vi "Main_Server.vi"() -> ()   [LabVIEW 2013]
uses:
  Control/TCP Multiple Connections Data.ctl
  GlobleVar/port.vi
panel:
  in  "Data":T1
  out "error out":errorcluster
  out "Message Received":string[](array[string])
  out "To Client":string
  in  "stop":bool
  out "已连接的设备数量":u32
  out "已连接的设备":string[](array[string])
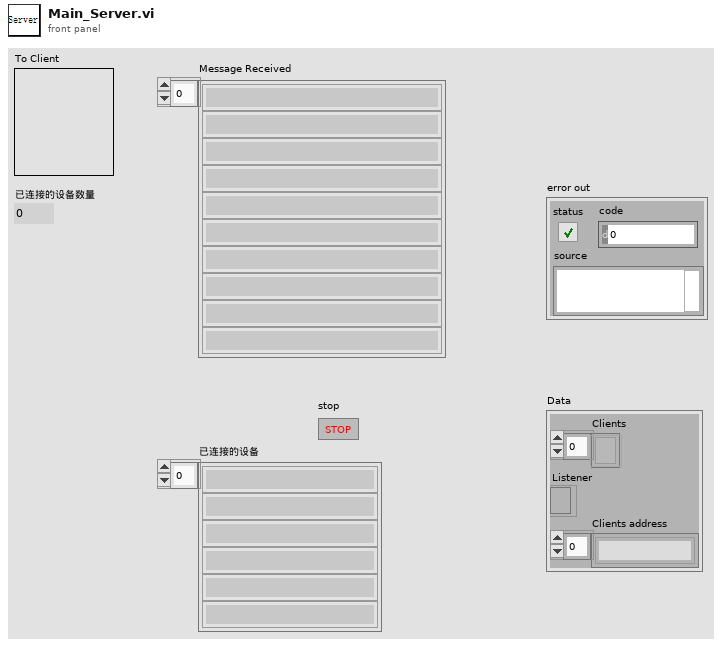
[diagram p1: front panel]
types:
  T1 = typedef "TCP Multiple Connections Data.ctl" = cluster{"Clients":refnum<k5>[], "Listener":refnum<k5>, "Clients address":string[]}
  T2 = cluster{"联机状态":bool, "外置清零信号":bool, "卡件工作模式":enum16{"无输出", "正常工作", "阀门常开", "阀门常闭"}, "卡件序列号":string, "卡件物理地址":string, "伺服阀输出电流CH1":dbl, "输出通道状态CH1":bool, "伺服阀输出电流CH2":dbl, "输出通道状态CH2":bool, "伺服输出使能CH1 ":bool, "伺服输出使能CH2":bool, "LVDT1类型":enum16{"未接入", "直流", "交流"}, "LVDT1直流回路":bool, "LVDT1次级线圈 2":bool, "LVDT1次级线圈 1":bool, "LVDT1初级线圈":bool, "LVDT2类型":enum16{"未接入", "直流", "交流"}, "LVDT2直流回路":bool, "LVDT2次级线圈 2":bool, "LVDT2次级线圈 1":bool, "LVDT2初级线圈":bool, "DEH回路状态":bool, "DEH类型":enum16{"内置", "外接"}, "转速反馈使能":bool, "LVDT1信号采样百分比":dbl, "LVDT2信号采样百分比":dbl, "DEH指令值":u8, "转速差反馈量":dbl, "回路1转速":dbl, "回路2转速":dbl, "回路3转速":dbl, "中选转速":dbl, "LVDT1 ADC":i16, "LVDT2 ADC":i16, "DEH ADC":i16, "LVDT1ZADC":i16, "LVDT2ZADC":i16, "LVDT1FADC":i16, "LVDT2FADC":i16, "DehZeroCali":bool, "DehFullCali":bool, "LVDT1ZeroCali":bool, "LVDT1FullCali":bool, "LVDT2ZeroCali":bool, "LVDT2FullCali":bool, "转速零度标定":i16, "转速满度标定":i16, "转速指令采样值":i16, "标准转速":dbl}
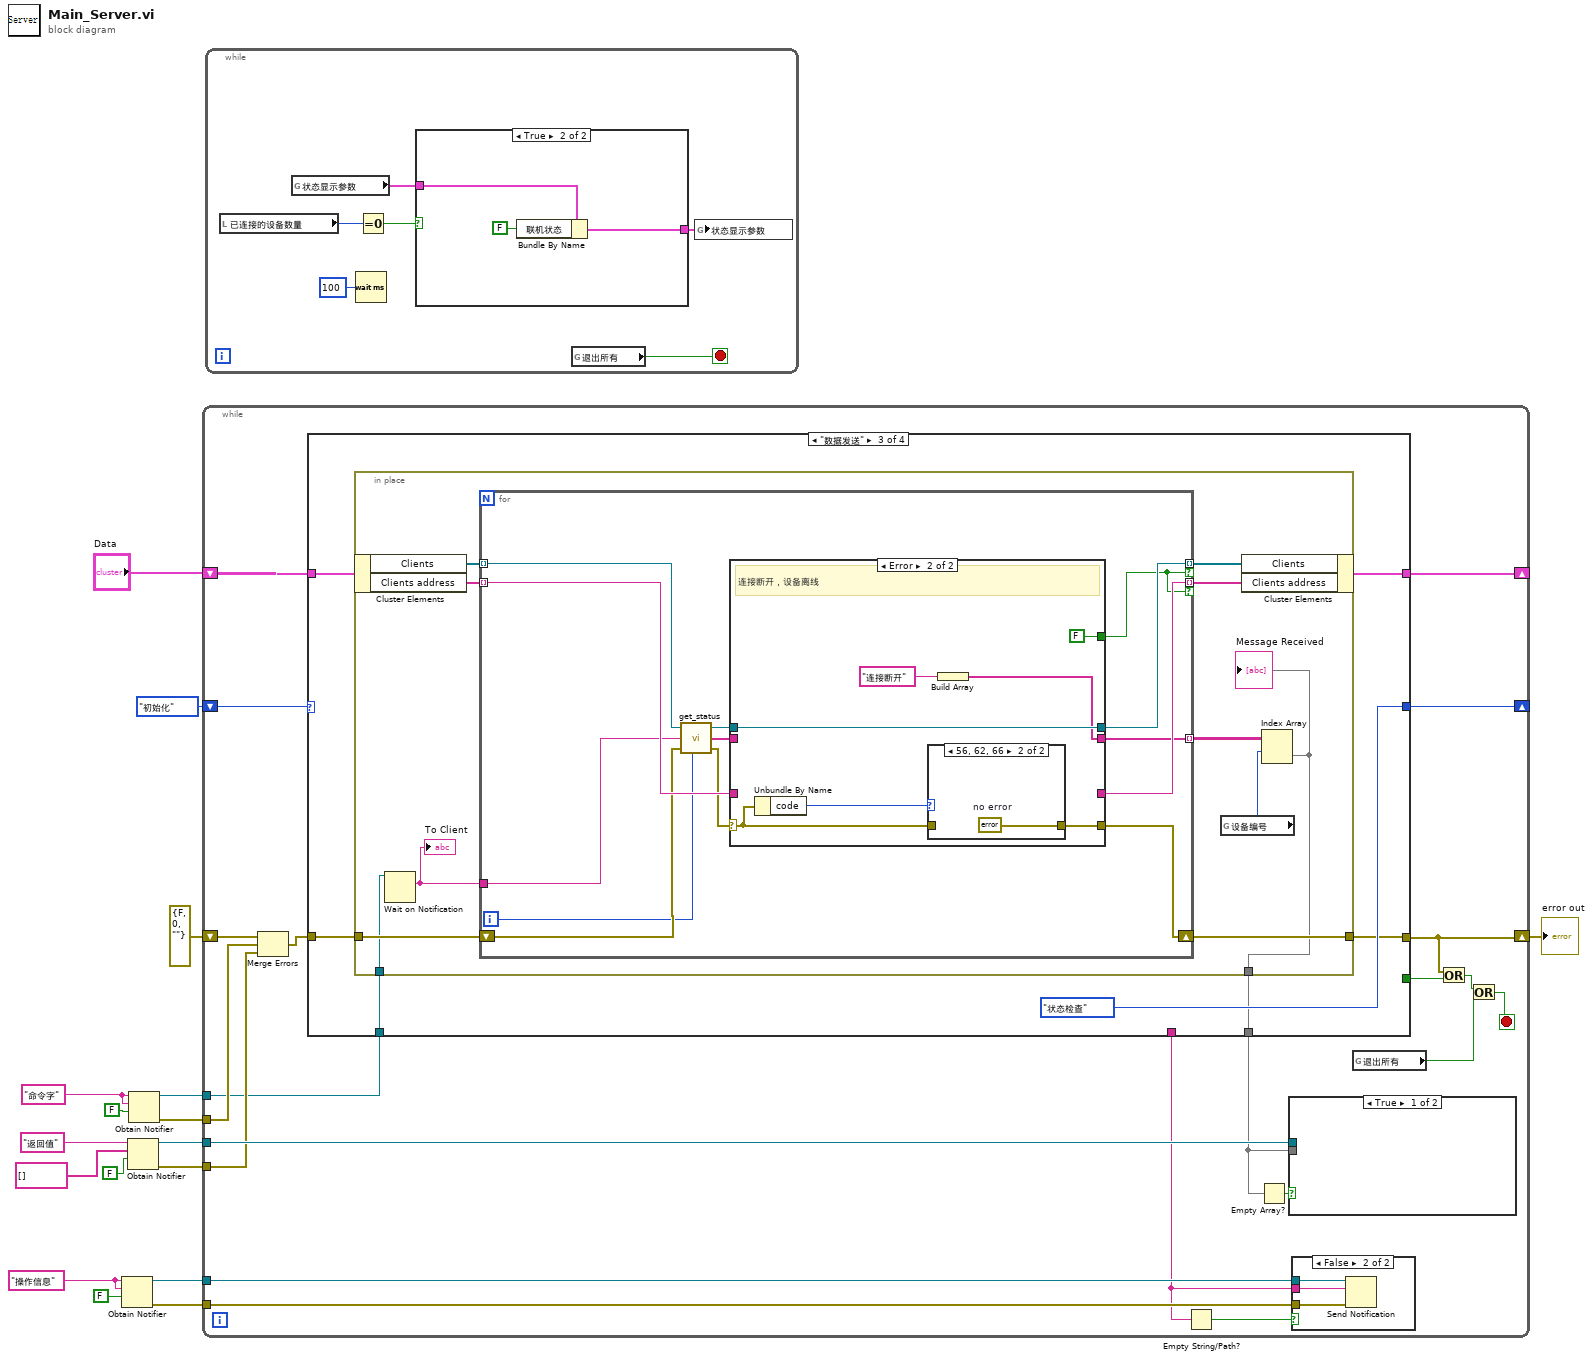
[diagram p0: block diagram]
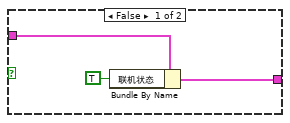
[diagram p2: hidden frame]
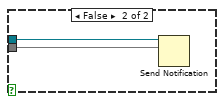
[diagram p4: hidden frame]
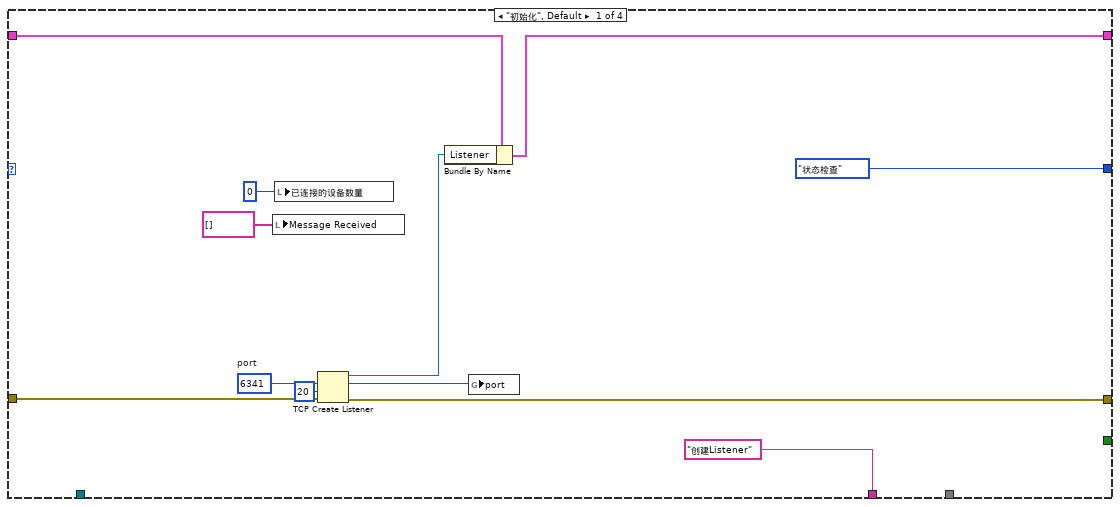
[diagram p5: hidden frame]
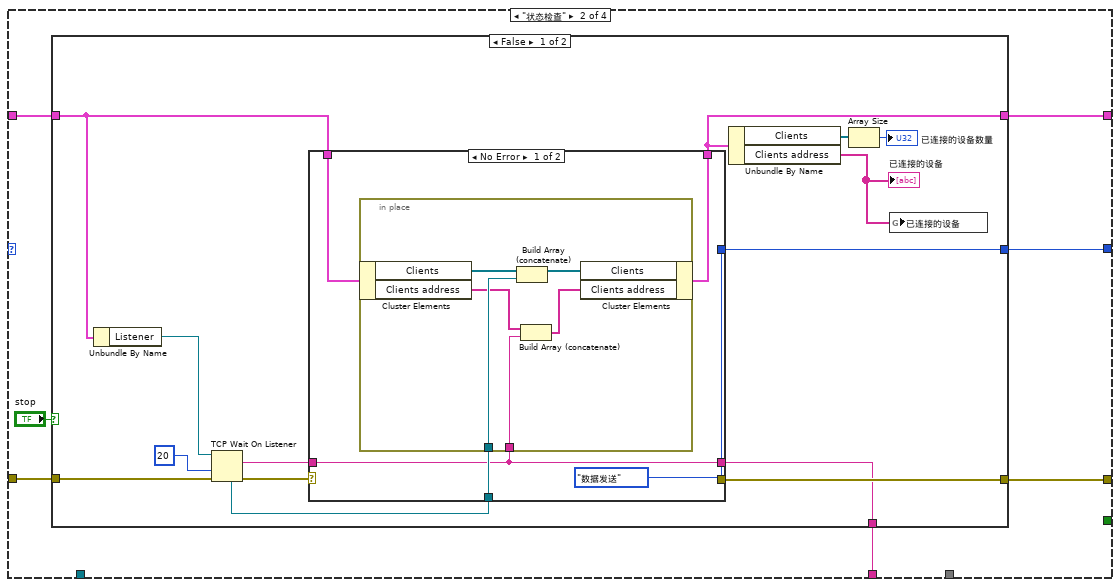
[diagram p6: hidden frame]
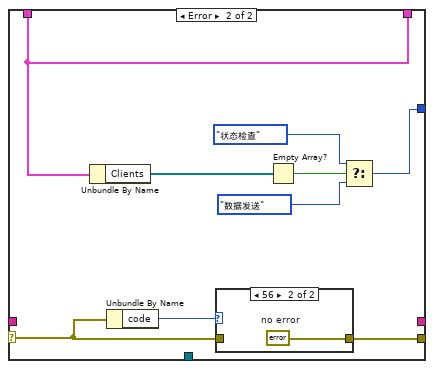
[diagram p7: hidden frame]
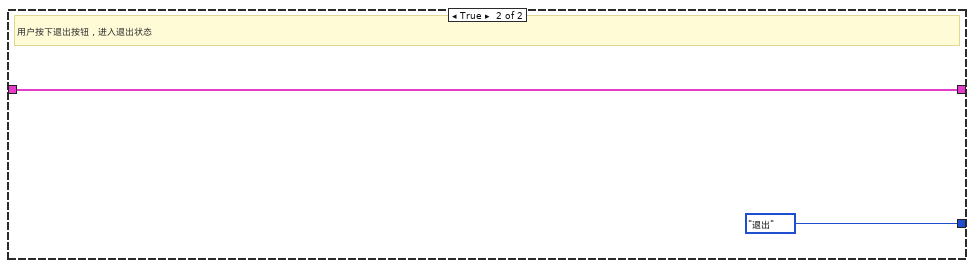
[diagram p9: hidden frame]
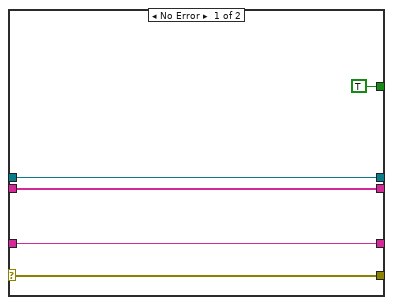
[diagram p10: hidden frame]
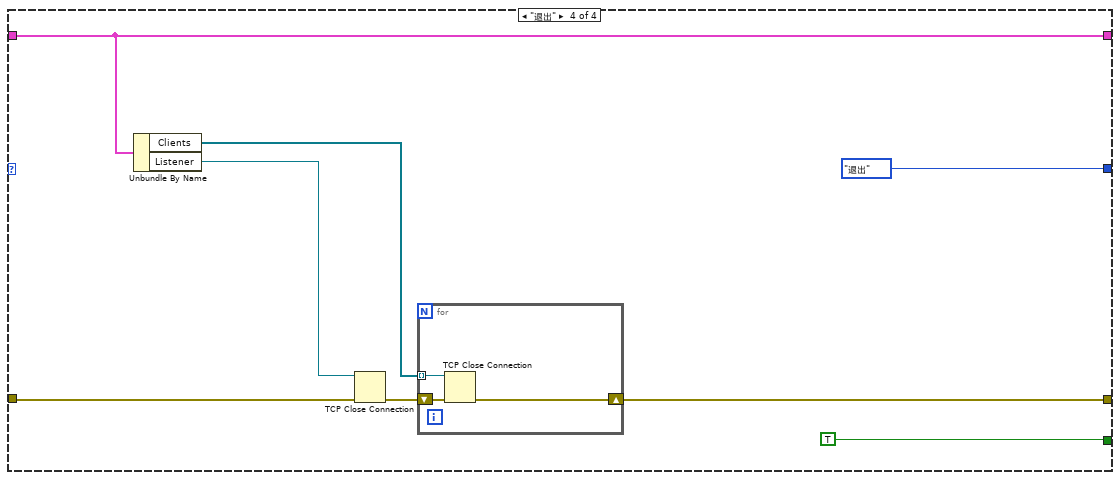
[diagram p12: hidden frame]
diagram:
  w4 = "操作信息"
  w10 = "命令字"
  n1 = Obtain Notifier(name (unnamed)=w4, notification data type=w4, create if not found? (T)=FALSE) -> (notifier out=w2:refnum<notifier>, error out=w1:errorcluster)  [unwired: 1 in, 1 out]
  n2 = Obtain Notifier(name (unnamed)="返回值", notification data type=string[] [], create if not found? (T)=FALSE) -> (notifier out=w8:refnum<notifier>, error out=w6:errorcluster)  [unwired: 1 in, 1 out]
  n3 = Obtain Notifier(name (unnamed)=w10, notification data type=w10, create if not found? (T)=FALSE) -> (notifier out=w7:refnum<notifier>, error out=w5:errorcluster)  [unwired: 1 in, 1 out]
  n4 = while {
    shift-right: [w37] -> _
    shift-left: enum16{"初始化", "状态检查", "数据发送", "退出"}."初始化" -> [w38]
    shift-right: [w33] -> _
    shift-left: "Data" -> [w36]
    shift-right: [w34] -> w14
    shift-left: errorcluster {"status"=FALSE, "code"=0, "source"=""} ("error out") -> [w26]
    tunnel: w8 -> [w31]
    tunnel: w7 -> [w18]
    tunnel: w6 -> [w23]
    tunnel: w5 -> [w25]
    tunnel: w2 -> [w21]
    tunnel: w1 -> [w20]
    stop <- w27 stop-if-true
    n5 = Merge Errors(w26, w25, w23) -> (w24:errorcluster)
    n6 = case shown="\"数据发送\"" w38 {
      tunnel: [enum16{"初始化", "状态检查", "数据发送", "退出"}."状态检查" w61 enum16{"初始化", "状态检查", "数据发送", "退出"}."状态检查" enum16{"初始化", "状态检查", "数据发送", "退出"}."退出"] -> w37
      tunnel: w24 -> [w52 w59 w104 w151]
      tunnel: [w51 w57 w103 w152] -> w34
      tunnel: w36 -> [w49 w60 w106 w147]
      tunnel: [w50 w58 w105 w147] -> w33
      tunnel: [_ _ _ TRUE] -> w35
      tunnel: [_ _ w102 _] -> w30
      tunnel: ["创建Listener" w56 _ _] -> w19
      tunnel: w18 -> [_ _ w101 _]
      frame "初始化", Default {
        w54 = u16 6341  # port
        n7 = local write "Message Received"(string[] [] ("Message Received")) -> ()
        n8 = local write "已连接的设备数量"(u32 0 ("已连接的设备数量")) -> ()
        n9 = TCP Create Listener(8:w52, 9:20 ("timeout ms (25000)"), 10:w54) -> (0:w51:errorcluster, 2:w46:u16, 3:w53:refnum<k5>)  [unwired: 2 out]
        n10 = Bundle By Name(cluster=w49, "Listener"=w53) -> (w50:T1)
        n11 = global write "port.vi" "port"(w46) -> ()
      }
      frame "状态检查" {
        n12 = case shown="False" "stop" {
          tunnel: [w69 enum16{"初始化", "状态检查", "数据发送", "退出"}."退出"] -> w61
          tunnel: w60 -> [w73 w99]
          tunnel: w59 -> [w75 _]
          tunnel: [w67 w99] -> w58
          tunnel: [w68 _] -> w57
          tunnel: [w63 _] -> w56
          frame False {
            n13 = Unbundle By Name(w73) -> ("Listener"=w76:refnum<k5>)
            n14 = TCP Wait On Listener(8:w75, 9:20 ("timeout ms (wait forever: -1)"), 11:w76) -> (0:w74:errorcluster, 2:w71:string, 4:w72:refnum<k5>)  [unwired: 1 in, 2 out]
            n15 = case shown="No Error" w74 {
              selector: w74 -> [_ w88]
              tunnel: w73 -> [w81 w91]
              tunnel: w72 -> [w80 _]
              tunnel: w71 -> [w77 _]
              tunnel: [w78 w91] -> w67
              tunnel: [enum16{"初始化", "状态检查", "数据发送", "退出"}."数据发送" w92] -> w69
              tunnel: [_ w89] -> w68
              tunnel: [w77 _] -> w63
              frame No Error {
                n16 = in-place {
                  in-place-border: w80 -> [w86]
                  in-place-border: w77 -> [w85]
                  n17 = in-place-cluster #1(w81) -> ("Clients"=w87:refnum<k5>[], "Clients address"=w83:string[])
                  n18 = Build Array (concatenate)(w87, w86) -> (w84:refnum<k5>[])
                  n19 = Build Array (concatenate)(w83, w85) -> (w82:string[])
                  n20 = in-place-cluster #1("Clients"=w84, "Clients address"=w82) -> (w78:T1)
                }
              }
              frame Error {
                n21 = Unbundle By Name(w91) -> ("Clients"=w96:refnum<k5>[])
                n22 = Unbundle By Name(w88) -> ("code"=w90:i32)
                n23 = case shown="56" w90 {
                  tunnel: [w97 w98] -> w89
                  tunnel: w88 -> [w97 _]
                  frame Default {
                  }
                  frame 56 {
                    w98 = errorcluster {"status"=FALSE, "code"=0, "source"=""}  # no error
                  }
                }
                n24 = Empty Array?(array=w96) -> (empty?=w95:bool)
                n25 = Select(t=enum16{"初始化", "状态检查", "数据发送", "退出"}."状态检查", s=w95, f=enum16{"初始化", "状态检查", "数据发送", "退出"}."数据发送") -> (s? t:f=w92:enum16{"初始化", "状态检查", "数据发送", "退出"})
              }
            }
            n26 = Unbundle By Name(w67) -> ("Clients"=w66:refnum<k5>[], "Clients address"=w64:string[])
            "已连接的设备" <- w64
            n27 = Array Size(array=w66) -> (size(s)=→"已连接的设备数量":i32)
            n28 = global write "已连接的设备.vi" "已连接的设备"(w64) -> ()
          }
          frame True {
            # "用户按下退出按钮，进入退出状态"
          }
        }
      }
      frame "数据发送" {
        n29 = in-place {
          in-place-border: w104 -> [w114]
          in-place-border: [w113] -> w103
          in-place-border: [w110] -> w102
          in-place-border: w101 -> [w109]
          n30 = in-place-cluster #2(w106) -> ("Clients"=w118:refnum<k5>[], "Clients address"=w115:string[])
          n31 = Wait on Notification(notifier=w109) -> (notification=w108:string)  [unwired: 3 in, 3 out]
          "To Client" <- w108
          n32 = for {
            tunnel: w118 -> [w131] mode=indexing
            tunnel: [w130] -> w117 mode=indexing if=w126
            tunnel: [w129] -> w116 mode=indexing if=w126
            tunnel: w115 -> [w128] mode=indexing
            shift-right: [w127] -> w113
            shift-left: w114 -> [w125]
            tunnel: [w124] -> w112 mode=indexing
            tunnel: w108 -> [w120]
            i -> [w119]
            n33 = call "get_status.vi"("connection ID in"=w131, "command in"=w120, "error in"=w125, "设备编号"=w119) -> ("connection ID out"=w122:refnum<k5>, "Status received"=w123:string[], "error out"=w121:errorcluster)  [unwired: 1 in]
            n34 = case shown="Error" w121 {
              selector: w121 -> [w136 w141]
              tunnel: [w136 w142] -> w127
              tunnel: w123 -> [w132 _]
              tunnel: w122 -> [w135 w140]
              tunnel: [w135 w140] -> w130
              tunnel: w128 -> [w134 _]
              tunnel: [w134 _] -> w129
              tunnel: [TRUE FALSE] -> w126
              tunnel: [w132 w138] -> w124
              frame No Error {
              }
              frame Error {
                # "连接断开，设备离线"
                n35 = Unbundle By Name(w141) -> ("code"=w143:i32)
                n36 = case shown="56, 62, 66" w143 {
                  tunnel: [w144 w145] -> w142
                  tunnel: w141 -> [w144 _]
                  frame Default {
                  }
                  frame 56, 62, 66 {
                    w145 = errorcluster {"status"=FALSE, "code"=0, "source"=""}  # no error
                  }
                }
                n37 = Build Array("连接断开") -> (w138:string[])
              }
            }
          }
          n38 = global read "设备编号.vi" "设备编号"() -> (w111:u8)
          n39 = in-place-cluster #2("Clients"=w117, "Clients address"=w116) -> (w105:T1)
          n40 = Index Array(array=w112, index (row)=w111) -> (element=w110:string[])  [unwired: 1 in]
          "Message Received" <- w110
        }
      }
      frame "退出" {
        n41 = Unbundle By Name(w147) -> ("Clients"=w149:refnum<k5>[], "Listener"=w150:refnum<k5>)
        n42 = TCP Close Connection(connection ID=w150, error in (no error)=w151) -> (error out=w153:errorcluster)  [unwired: 1 in, 1 out]
        n43 = for {
          shift-right: [w155] -> w152
          shift-left: w153 -> [w156]
          tunnel: w149 -> [w154] mode=indexing
          n44 = TCP Close Connection(connection ID=w154, error in (no error)=w156) -> (error out=w155:errorcluster)  [unwired: 1 in, 1 out]
        }
      }
    }
    n45 = Empty String/Path?(string/path=w19) -> (empty?=w22:bool)
    n46 = Empty Array?(array=w30) -> (empty?=w32:bool)
    n47 = case shown="True" w32 {
      tunnel: w31 -> [_ w43]
      tunnel: w30 -> [_ w42]
      frame True {
      }
      frame False {
        n48 = Send Notification(notification=w42, notifier=w43) -> ()  [unwired: 1 in, 2 out]
      }
    }
    n49 = case shown="False" w22 {
      tunnel: w21 -> [_ w41]
      tunnel: w20 -> [_ w40]
      tunnel: w19 -> [_ w39]
      frame True {
      }
      frame False {
        n50 = Send Notification(notification=w39, notifier=w41, error in (no error)=w40) -> ()  [unwired: 2 out]
      }
    }
    n51 = global read "退出所有.vi" "退出所有"() -> (w28:bool)
    n52 = Or(x=w34, y=w35) -> (x .or. y?=w29:bool)
    n53 = Or(x=w29, y=w28) -> (x .or. y?=w27:bool)
  }
  "error out" <- w14
  n54 = while {
    stop <- w162 stop-if-true
    n55 = local read "已连接的设备数量"() -> (w161:u32)
    n56 = global read "状态显示参数.vi" "状态显示参数"() -> (w158:T2)
    n57 = Wait (ms)(milliseconds to wait=u32 100) -> ()  [unwired: 1 out]
    n58 = Equal To 0?(x=w161) -> (x = 0?=w159:bool)
    n59 = case shown="True" w159 {
      tunnel: w158 -> [w164 w167]
      tunnel: [w163 w166] -> w157
      frame False {
        n60 = Bundle By Name(cluster=w164, "联机状态"=TRUE) -> (w163:T2)
      }
      frame True {
        n61 = Bundle By Name(cluster=w167, "联机状态"=FALSE) -> (w166:T2)
      }
    }
    n62 = global read "退出所有.vi" "退出所有"() -> (w162:bool)
    n63 = global write "状态显示参数.vi" "状态显示参数"(w157) -> ()
  }
